vi "Write Steering Frame.vi"(6 "Teleop command":T1, 8 "error in (no error)":errorcluster, 11 "ROV in":refnum<class "ROV Host.lvclass">) -> (0 "error out":errorcluster, 3 "ROV out":refnum<class "ROV Host.lvclass">)   [LabVIEW 2012, in "ROV Host.lvclass"]
doc: "This VI is used to assign a new frame velocity to the drivetrains using the generated or received teleop command.\nRuffin"
uses:
  ROV Host.lvclass
  Teleop command.ctl
  ROV Host.lvclass/ROV Host.ctl
  <vilib>/robotics/Steering/Steering Frame/NI_Robotics_Steering Frame.lvclass/NI_Robotics_Steering Frame.ctl
  Support/Host globals (robot acquires video).vi
  <vilib>/robotics/Steering/Steering Frame/Get Steering Frame Velocity from Wheels.vi
  <vilib>/robotics/Steering/Steering Frame/NI_Robotics_Steering Frame.lvclass
  <vilib>/robotics/Steering/Steering Frame/Get Steering Frame Velocity from Motors.vi
  <vilib>/robotics/Steering/Steering Frame/Apply Steering Frame Velocity to Wheels.vi
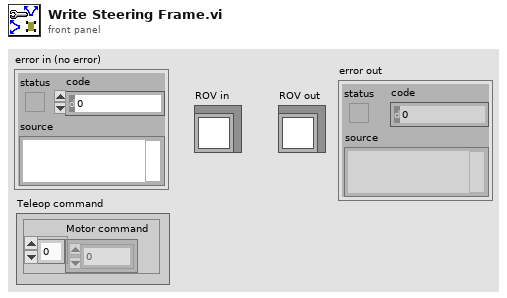
[diagram p1: front panel]
types:
  T1 = typedef "ROV Host.lvclass/Teleop command.ctl" = cluster{"Motor command":i8[]}
  T2 = typedef "NI_Robotics_Steering Class Types.lvlib/Mecanum Steering Frame.ctl" = refnum<class "NI_Robotics_Mecanum Steering Frame.lvclass">
  T3 = typedef "NI_Robotics_Steering Class Types.lvlib/Differential Steering Frame.ctl" = refnum<class "NI_Robotics_Differential Steering Frame.lvclass">
  T4 = typedef "NI_Robotics_Wheel.lvclass/Wheel State.ctl" = cluster{"wheel name":string, "forward angular velocity":dbl, "caster angular velocity":dbl, "caster wheel angle (rad)":dbl, "steering angle (rad)":dbl}
  T5 = cluster{"mecanum steering frame out":T2, "differential steering frame out":T3}
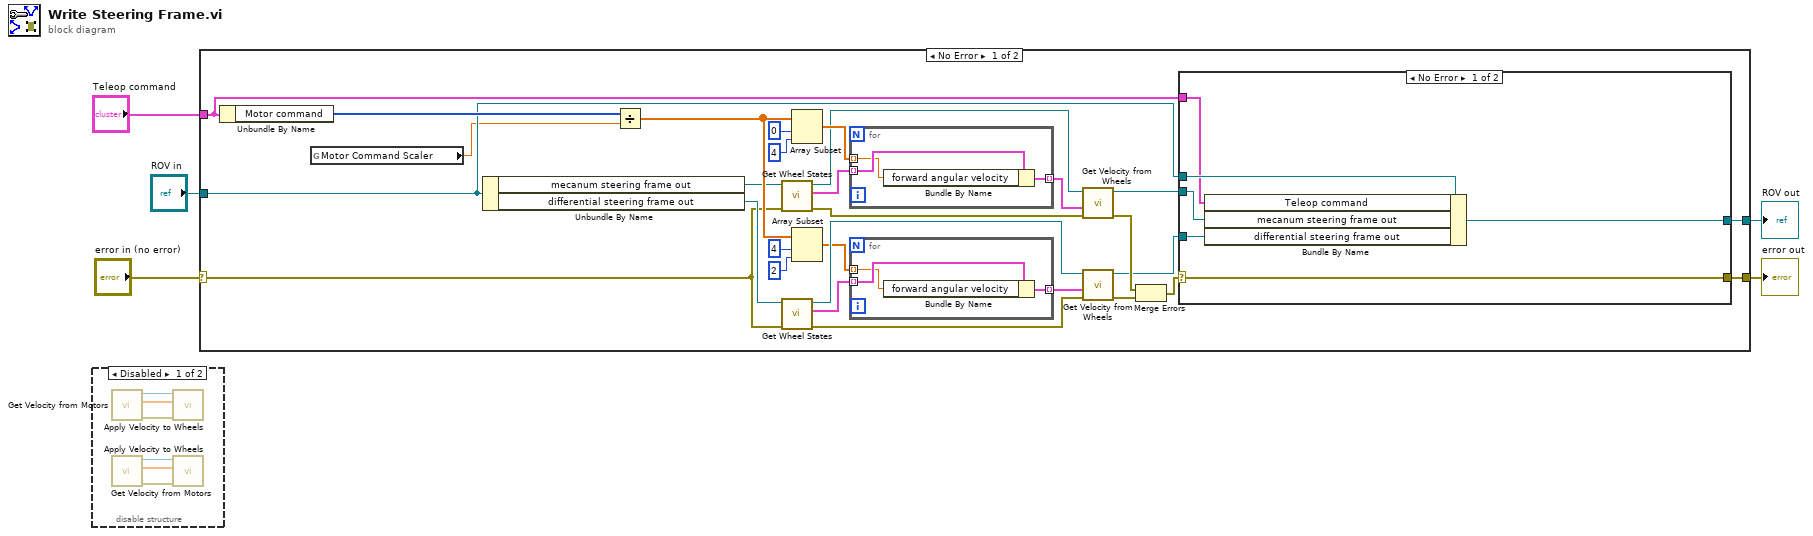
[diagram p0: block diagram]
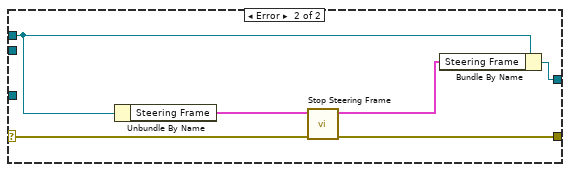
[diagram p3: hidden frame]
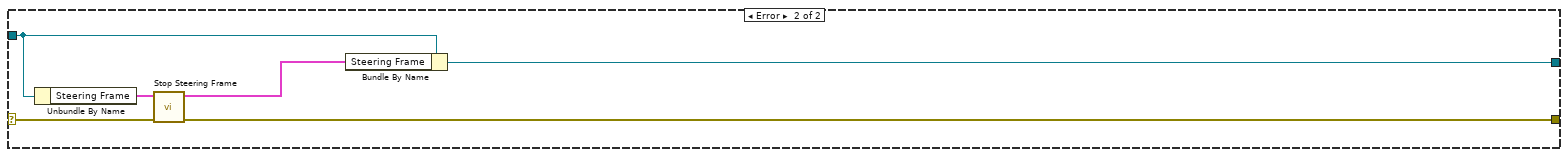
[diagram p4: hidden frame]
diagram:
  n1 = disable-structure shown="Disabled" {
    frame Disabled {
      n2 = call-poly <vilib>:"Get Velocity from Motors.vi"() -> ("error out"=w9:errorcluster, "estimated steering frame velocity"=w10:dbl[], "steering frame out"=w11:refnum<class "NI_Robotics_Steering Frame.lvclass">)  [unwired: 9 in]
      n3 = call-poly <vilib>:"Get Velocity from Motors.vi"() -> ("error out"=w8:errorcluster, "estimated steering frame velocity"=w6:dbl[], "steering frame out"=w7:refnum<class "NI_Robotics_Steering Frame.lvclass">)  [unwired: 9 in]
      n4 = call-poly <vilib>:"Apply Velocity to Wheels.vi"("error in (no error)"=w9, "steering frame velocity"=w10, "steering frame in"=w11) -> ("error out"=w13:errorcluster)  [unwired: 5 in, 3 out]
      n5 = call-poly <vilib>:"Apply Velocity to Wheels.vi"("error in (no error)"=w8, "steering frame velocity"=w6, "steering frame in"=w7) -> ("error out"=w12:errorcluster)  [unwired: 5 in, 3 out]
    }
    frame Enabled {
    }
  }
  n6 = case shown="No Error" "error in (no error)" {
    selector: "error in (no error)" -> [w18 w66]
    tunnel: [w33 w65] -> w4
    tunnel: "Teleop command" -> [w35 _]
    tunnel: "ROV in" -> [w34 w62]
    tunnel: [w32 w61] -> w1
    frame No Error {
      n7 = Unbundle By Name(w35) -> ("Motor command"=w38:i8[])
      n8 = global read "Host globals (robot acquires video).vi" "Motor Command Scaler"() -> (w14:dbl)
      n9 = Unbundle By Name(w34) -> ("mecanum steering frame out"=w31:T2, "differential steering frame out"=w19:T3)
      n10 = Divide(x=w38, y=w14) -> (x/y=w37:dbl[])
      n11 = call <vilib>:"Get Wheel States.vi"("error in (no error)"=w18, "steering frame in"=w31) -> ("error out"=w27:errorcluster, "wheel states"=w30:T4[], "steering frame out"=w26:T2)  [unwired: 7 in]
      n12 = call <vilib>:"Get Wheel States.vi"("error in (no error)"=w18, "steering frame in"=w19) -> ("error out"=w16:errorcluster, "wheel states"=w22:T4[], "steering frame out"=w21:T3)  [unwired: 7 in]
      n13 = Array Subset(array=w37, index=0, length=4) -> (w29:dbl[])
      n14 = Array Subset(array=w37, index=4, length=2) -> (w15:dbl[])
      n15 = for {
        tunnel: w30 -> [w48] mode=indexing
        tunnel: w29 -> [w47] mode=indexing
        tunnel: [w46] -> w28 mode=indexing
        n16 = Bundle By Name(cluster=w48, "forward angular velocity"=w47) -> (w46:T4)
      }
      n17 = for {
        tunnel: w22 -> [w45] mode=indexing
        tunnel: w15 -> [w44] mode=indexing
        tunnel: [w43] -> w23 mode=indexing
        n18 = Bundle By Name(cluster=w45, "forward angular velocity"=w44) -> (w43:T4)
      }
      n19 = call-poly <vilib>:"Get Velocity from Wheels.vi"("error in (no error)"=w27, "acquired wheel states"=w28, "steering frame in"=w26) -> ("error out"=w24:errorcluster, "steering frame out"=w25:T2)  [unwired: 5 in, 2 out]
      n20 = call-poly <vilib>:"Get Velocity from Wheels.vi"("error in (no error)"=w16, "acquired wheel states"=w23, "steering frame in"=w21) -> ("error out"=w17:errorcluster, "steering frame out"=w20:T3)  [unwired: 5 in, 2 out]
      n21 = Merge Errors(w24, w17) -> (w36:errorcluster)
      n22 = case shown="No Error" w36 {
        selector: w36 -> [w52 w57]
        tunnel: w35 -> [w51 _]
        tunnel: w34 -> [w54 w58]
        tunnel: [w52 w56] -> w33
        tunnel: [w53 w55] -> w32
        tunnel: w25 -> [w50 _]
        tunnel: w20 -> [w49 _]
        frame No Error {
          n23 = Bundle By Name(cluster=w54, "Teleop command"=w51, "mecanum steering frame out"=w50, "differential steering frame out"=w49) -> (w53:refnum<class "ROV Host.lvclass">)
        }
        frame Error {
          n24 = Unbundle By Name(w58) -> ("Steering Frame"=w59:T5)
          n25 = call "Stop Steering Frame.vi"("error in (no error)"=w57, "Steering Frame in"=w59) -> ("error out"=w56:errorcluster, "Steering Frame out"=w60:T5)  [unwired: 8 in]
          n26 = Bundle By Name(cluster=w58, "Steering Frame"=w60) -> (w55:refnum<class "ROV Host.lvclass">)
        }
      }
    }
    frame Error {
      n27 = Unbundle By Name(w62) -> ("Steering Frame"=w63:T5)
      n28 = call "Stop Steering Frame.vi"("error in (no error)"=w66, "Steering Frame in"=w63) -> ("error out"=w65:errorcluster, "Steering Frame out"=w64:T5)  [unwired: 8 in]
      n29 = Bundle By Name(cluster=w62, "Steering Frame"=w64) -> (w61:refnum<class "ROV Host.lvclass">)
    }
  }
  "error out" <- w4
  "ROV out" <- w1
